vi "EntireSpectrumProcess.vi"(11 "data":waveform(dbl)) -> (1 "RMS":dynamicdata(waveform), 2 "Dynamic Data":dynamicdata(waveform), 3 "Array":cluster{dbl, dbl}[](array[cluster]))   [LabVIEW 2017]
uses:
  <vilib>/Analysis/NI_AALPro.lvlib
  <vilib>/Analysis/2dsp.llb/Real FFT.vi
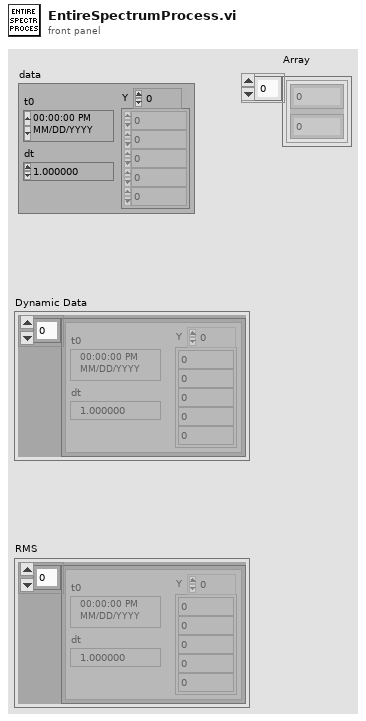
[diagram p1: front panel]
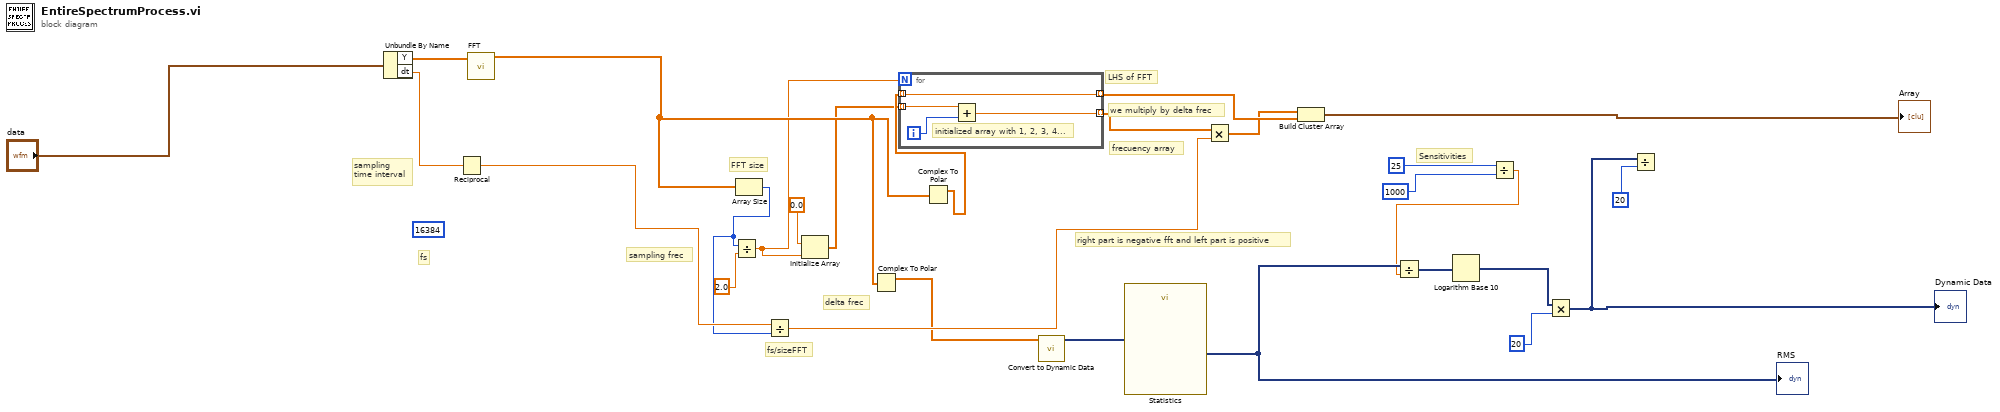
[diagram p0: block diagram]
diagram:
  (unwired) 16384
  # "LHS of FFT"
  # "frecuency array"
  # "delta frec"
  # "we multiply by delta frec"
  # "fs/sizeFFT"
  # "sampling frec"
  # "FFT size"
  # "right part is negative fft and left part is positive"
  # "Sensitivities"
  # "sampling \ntime interval"
  # "fs"
  n1 = Unbundle By Name("data") -> ("Y"=w1:dbl[], "dt"=w2:dbl)
  n2 = Reciprocal(x=w2) -> (1/x=w26:dbl)
  n3 = call-poly <vilib>:"FFT.vi"("X"=w1) -> ("FFT {X}"=w25:cdb[])  [unwired: 9 in, 1 out]
  n4 = Array Size(array=w25) -> (size(s)=w18:i32)
  n5 = Divide(x=w18, y=2.0) -> (x/y=w16:dbl)
  n6 = Divide(x=w26, y=w18) -> (x/y=w19:dbl)
  n7 = Initialize Array(0.0 ("element"), w16) -> (w17:dbl[])
  n8 = Complex To Polar(r * e^(i*theta)=w25) -> (r=w4:dbl[])  [unwired: 1 out]
  n9 = Complex To Polar(r * e^(i*theta)=w25) -> (r=w24:dbl[])  [unwired: 1 out]
  n10 = for {
    N: w16 -> [_]
    tunnel: w17 -> [w31] mode=indexing
    tunnel: [w29] -> w20 mode=indexing
    tunnel: w24 -> [w28] mode=indexing
    tunnel: [w28] -> w22 mode=indexing
    i -> [w30]
    # "initialized array with 1, 2, 3, 4..."
    n11 = Add(x=w31, y=w30) -> (x+y=w29:dbl)
  }
  n12 = call "Convert to Dynamic Data"("Array"=w4) -> ("Dynamic Data Type"=w3:dynamicdata)  [unwired: 3 in]
  n13 = call "Statistics"("Signals"=w3) -> ("RMS"=w8:dynamicdata)  [unwired: 25 in, 1 out]
  "RMS" <- w8
  n14 = Multiply(x=w20, y=w19) -> (x*y=w21:dbl[])
  n15 = Build Cluster Array(w21, w22) -> (→"Array":cluster{dbl, dbl}[])
  n16 = Divide(x=25, y=1000) -> (x/y=w7:dbl)
  n17 = Divide(x=w8, y=w7) -> (x/y=w9:dynamicdata)
  n18 = Logarithm Base 10(1:w9) -> (0:w10:dynamicdata)
  n19 = Multiply(x=w10, y=20) -> (x*y=w13:dynamicdata)
  "Dynamic Data" <- w13
  n20 = Divide(x=w13, y=20) -> ()  [unwired: 1 out]
